vi "GetEncoderData.vi"(8 "error in (no error)":errorcluster) -> (0 "error out":errorcluster, 2 "Encoder Data":T1)   [LabVIEW 2016, in "DriveBase.lvclass"]
uses:
  DriveBase.lvclass
  DriveBase.lvclass/DriveBase.ctl
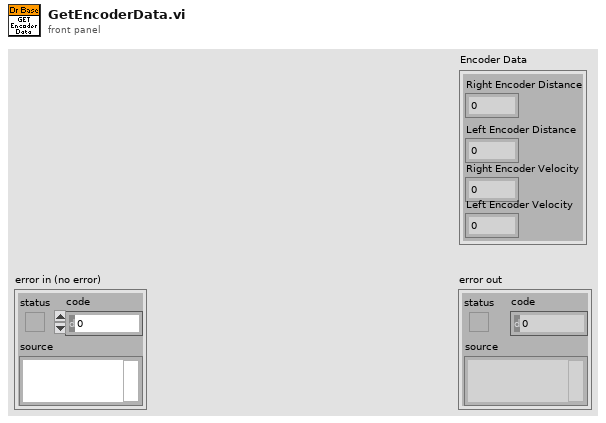
[diagram p1: front panel]
types:
  T1 = cluster{"Right Encoder Distance":dbl, "Left Encoder Distance":dbl, "Right Encoder Velocity":dbl, "Left Encoder Velocity":dbl}
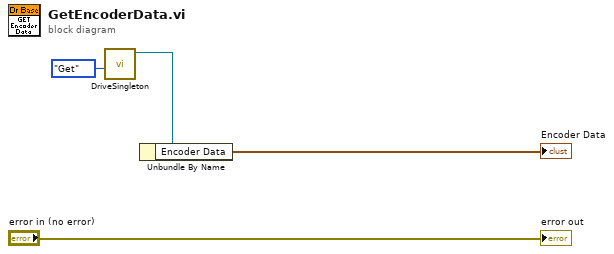
[diagram p0: block diagram]
diagram:
  n1 = call "DriveSingleton.vi"("Get/Set"=enum16{"Get", "Set"}."Get") -> ("DriveBase.lvclass 2"=w1:refnum<class "DriveBase.lvclass">)  [unwired: 9 in, 1 out]
  n2 = Unbundle By Name(w1) -> ("Encoder Data"=→"Encoder Data":T1)
  "error out" <- "error in (no error)"
